vi "Connect Newport Instrument_edit.vi"(4 "XON/XOFF (False)":bool, 6 "Baud Rate (921600 - USB)":u32=921600 min=300 max=115200 step=300, 7 "Filter Term for Instruments (\"\" - none)":string, 8 "error in (no error)":errorcluster, 10 "Numeric":i8, 11 "String":string) -> (0 "error (duplicate)":errorcluster, 1 "Connected":bool, 2 "VISA resource name (duplicate)":refnum<visa-resource-name>, 3 "Device Connection Cluster":T1, 5 "GPIB? ( T - GPIB, F - RS232 )":bool)   [LabVIEW 2014]
doc: "Connect Newport Device\n\nGet list of instrument, filter (if set) and allow for selection of device to talk to.\n\nThis is generic selection of the instrument to connected to, so look in system settings or on device to verify it is the correct port.\n\nInputs:\nFilter Term for Instruments (\"\" - none) - Term that will filter available displayed instruments based on term being in name, such as \"COM\".\n\nBaud Rate (921600 - USB) - Baud rate for serial communication\n\nXON/XOFF (False) - Sets whether XON/XOFF is used for serial communication.\n\nerror in - input error\n\nOutputs:\nGPIB? (T - GPIB, F - RS232) - Returns type of communication connected.\n\nConnected - Returns True if successful connection, False otherwise\n\nDevice Connection Cluster - Complete connection information for device, to be passed to communication VIs or Uncluster and pass only the VISA resource name, if that is all that is needed.\n\nVISA resource name (duplicate) - a copy of the name that is in Device Connection Cluster\n\nerror out (duplicate) - ouput error\n\nNOTE: \nFor SMC100, Input Baud Rate = 57600, Xon = True"
panel:
  # "s"
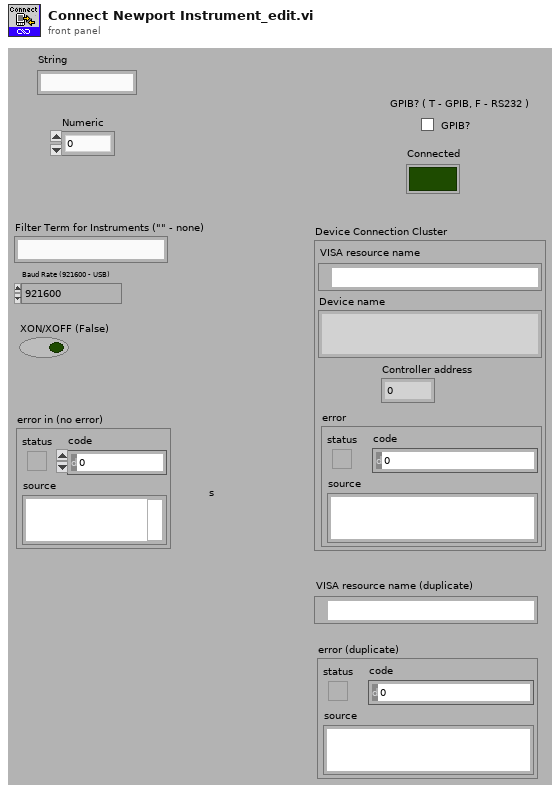
[diagram p1: front panel]
types:
  T1 = cluster{"VISA resource name":refnum<visa-resource-name>, "Device name":string, "Controller address":i32, "error":errorcluster}
  T2 = cluster{"VISA resource name":refnum<visa-resource-name>, "result string":string, "Controller address":i32, "error out":errorcluster}
  T3 = cluster{"VISA resource name":refnum<visa-resource-name>, "result string":string, "Numeric":i8, "error in (no error)":errorcluster}
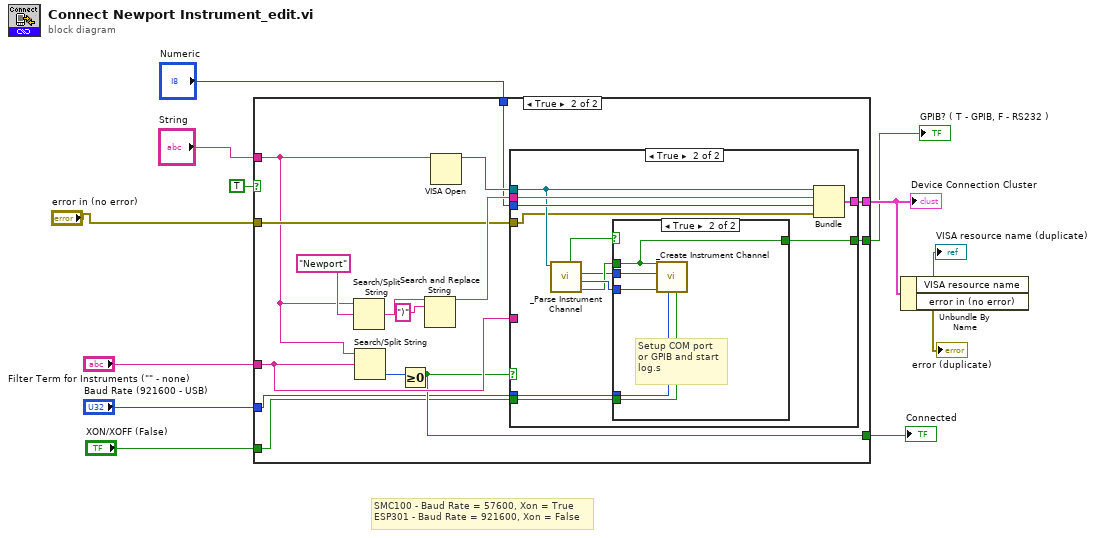
[diagram p0: block diagram]
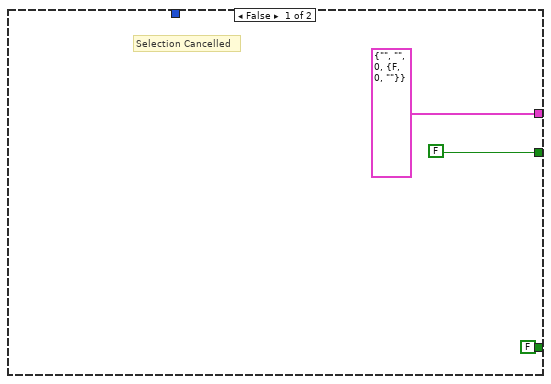
[diagram p2: hidden frame]
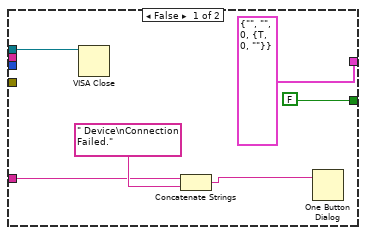
[diagram p3: hidden frame]
diagram:
  # "SMC100 - Baud Rate = 57600, Xon = True\nESP301 - Baud Rate = 921600, Xon = False"
  n1 = case shown="True" TRUE {
    tunnel: [T2 {"VISA resource name"="", "result string"="", "Controller address"=0, "error out"={"status"=FALSE, "code"=0, "source"=""}} w29] -> w8
    tunnel: "Filter Term for Instruments (\"\" - none)" -> [_ w23]
    tunnel: [FALSE w22] -> w11
    tunnel: "Baud Rate (921600 - USB)" -> [_ w21]
    tunnel: "XON/XOFF (False)" -> [_ w20]
    tunnel: [FALSE w19] -> w5
    tunnel: "String" -> [_ w16]
    tunnel: "Numeric" -> [_ w18]
    tunnel: "error in (no error)" -> [_ w17]
    frame False {
      # "Selection Cancelled"
    }
    frame True {
      n2 = Search/Split String(string=w16, search string/char (-)="Newport") -> (match + rest of string=w27:string)  [unwired: 1 in, 2 out]
      n3 = Search/Split String(string=w16, search string/char (-)=w23) -> (offset of match=w24:i32)  [unwired: 1 in, 2 out]
      n4 = Greater Or Equal To 0?(x=w24) -> (x >= 0?=w22:bool)
      n5 = Search and Replace String(input string=w27, search string=")") -> (result string=w25:string)  [unwired: 6 in, 3 out]
      n6 = VISA Open(VISA resource name=w16) -> (VISA resource name=w30:refnum<visa-resource-name>)  [unwired: 4 in, 1 out]
      n7 = case shown="True" w22 {
        tunnel: w30 -> [w35 w45]
        tunnel: w18 -> [_ w48]
        tunnel: [T2 {"VISA resource name"="", "result string"="", "Controller address"=0, "error out"={"status"=TRUE, "code"=0, "source"=""}} w47] -> w29
        tunnel: w25 -> [_ w46]
        tunnel: w23 -> [w32 _]
        tunnel: w21 -> [_ w41]
        tunnel: w20 -> [_ w38]
        tunnel: [FALSE w39] -> w19
        tunnel: w17 -> [_ w37]
        frame False {
          n8 = VISA Close(VISA resource name=w35) -> ()  [unwired: 1 in, 1 out]
          n9 = Concatenate Strings(w32, " Device\nConnection Failed." ("message")) -> (w34:string)
          n10 = One Button Dialog(message=w34) -> ()  [unwired: 1 in, 1 out]
        }
        frame True {
          n11 = call "_Parse Instrument Channel.vi"("Instrument Channel"=w45) -> ("T - GPIB, F - RS232"=w43:bool, "Hardware Address"=w44:i32, "Instrument Address"=w42:i16, "Valid String"=w40:bool)  [unwired: 6 in, 1 out]
          n12 = case shown="True" w40 {
            selector: w40 -> [w49 _]
            tunnel: w44 -> [_ w54]
            tunnel: w43 -> [_ w51]
            tunnel: w42 -> [_ w53]
            tunnel: w41 -> [_ w52]
            tunnel: [w49 w51] -> w39
            tunnel: w38 -> [_ w50]
            frame False {
            }
            frame True {
              # "Setup COM port\nor GPIB and start\nlog.s"
              n13 = call "_Create Instrument Channel.vi"("XON/XOFF (False)"=w50, "Baud Rate (921600 - USB)"=w52, "COM Port (1)"=w54, "GPIB Primary Address (4)"=w53, "(F), T - GPIB, F - RS232"=w51) -> ()  [unwired: 4 in, 3 out]
            }
          }
          n14 = Bundle("VISA resource name"=w45, "result string"=w46, "Numeric"=w48, "error in (no error)"=w37) -> (w47:T3)  [unwired: 1 in]
        }
      }
    }
  }
  "Device Connection Cluster" <- w8
  "Connected" <- w11
  "GPIB? ( T - GPIB, F - RS232 )" <- w5
  n15 = Unbundle By Name(w8) -> ("VISA resource name"=→"VISA resource name (duplicate)":refnum<visa-resource-name>, "error in (no error)"=→"error (duplicate)":errorcluster)
